vi "_FPGA Set LEDs.vi"(4 "error in (no error)":errorcluster, 5 "LED Command":T1) -> (0 "error out":errorcluster)   [LabVIEW 2015]
uses:
  Type/_LED States.ctl
  Type/_FPGA Indicator.ctl
  _RT Global.vi
  <vilib>/Utility/error.llb/Error Cluster From Error Code.vi
  <vilib>/rvi/errors/niLvFpgaAdjustHostInterfaceError.vi
  <vilib>/rvi/interface/nirviReadWriteControl/nirviReadWriteControl.xnode
  Type/FPGA Typedef.ctl
  FPGA Bitfiles/FPGA9607.lvbitx
  NiFpgaLv.dll
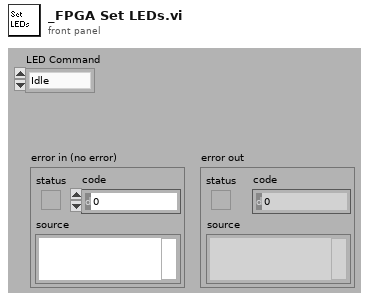
[diagram p1: front panel]
types:
  T1 = typedef "_LED States.ctl" = enum8{"Idle", "Solid B", "Solid R", "Solid P", "Off B", "Off R", "Off P", "Off BRP", "Off RP", "Flash R&P", "Flash P"}
  T2 = typedef "_FPGA Indicator.ctl" = enum16{"Done", "Ready", "Count Available", "SendSerial", "LED State"}
  T3 = typedef "FPGA Typedef.ctl" = refnum<k20>
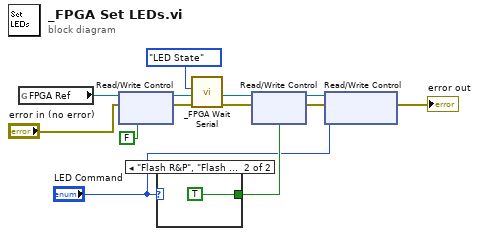
[diagram p0: block diagram]
diagram:
  n1 = global read "_RT Global.vi" "FPGA Ref"() -> (w2:T3)
  n2 = xnode "Read/Write Control"("FPGA VI Reference In"=w2, "error in"="error in (no error)", "Repeat"=FALSE ("Start")) -> ("FPGA VI Reference Out"=w1:T3, "error out"=w10:errorcluster)
  n3 = case shown="\"Flash R&P\", \"Flash P\"" "LED Command" {
    tunnel: [_ TRUE ("Start")] -> w7
    frame "Idle", Default {
    }
    frame "Flash R&P", "Flash P" {
    }
  }
  n4 = call "_FPGA Wait Serial.vi"("error in"=w10, "Indicator"=_FPGA_Indicator."LED State") -> ("error out"=w8:errorcluster)  [unwired: 3 in, 2 out]
  n5 = xnode "Read/Write Control"("FPGA VI Reference In"=w1, "error in"=w8, "Repeat"=w7) -> ("FPGA VI Reference Out"=w6:T3, "error out"=w5:errorcluster)
  n6 = xnode "Read/Write Control"("FPGA VI Reference In"=w6, "error in"=w5, "LED States"="LED Command") -> ("error out"=→"error out":errorcluster)  [unwired: 1 out]
